vi "ModeDrivebase.vi"(0 "Master State":enum16{"Normal", "Climb"}(ring)) -> (1 "Drive Mode Change":bool, 2 "Drive Mode":T1(ring))   [LabVIEW 2020]
doc: "This VI manages the robot drivebase mode. The default mode is driver control in which the swerve drive accepts all drive inputs and seemlessly combines them with autonomous heading corrections. Two auto targeting modes are also implimented."
uses:
  dscommands.vi
  dsdata.vi
  sensors.vi
  outputs.vi
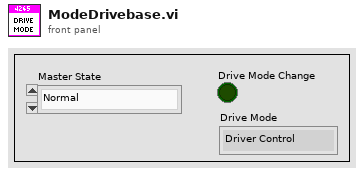
[diagram p1: front panel]
types:
  T1 = enum16{"Driver Control", "Auto Targeting", "Feeder Station"}
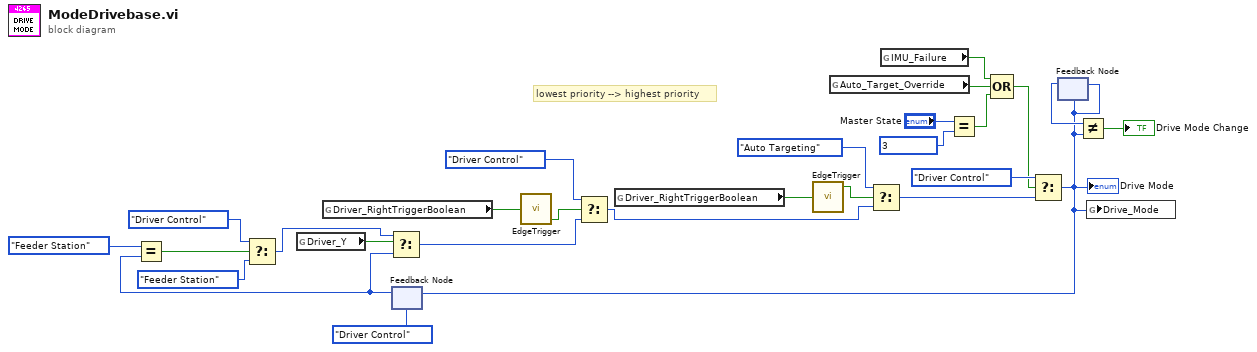
[diagram p0: block diagram]
diagram:
  # "lowest priority --> highest priority"
  n1 = global read "dscommands.vi" "Driver_Y"() -> (w14:bool)
  n2 = global read "dscommands.vi" "Driver_RightTriggerBoolean"() -> (w6:bool)
  n3 = feedback #1(T1."Driver Control") -> (w11:T1)
  n4 = Equal?(x=T1."Feeder Station", y=w11) -> (x = y?=w19:bool)
  n5 = Select(t=T1."Driver Control", s=w19, f=T1."Feeder Station") -> (s? t:f=w8:T1)
  n6 = Select(t=w8, s=w14, f=w11) -> (s? t:f=w4:T1)
  n7 = call "EdgeTrigger.vi"("Input Signal"=w6) -> ("Falling Edge Trigger"=w5:bool)  [unwired: 2 out]
  n8 = Select(t=T1."Driver Control", s=w5, f=w4) -> (s? t:f=w3:T1)
  n9 = global read "dscommands.vi" "Driver_RightTriggerBoolean"() -> (w10:bool)
  n10 = call "EdgeTrigger.vi"("Input Signal"=w10) -> ("Rising Edge Trigger"=w9:bool)  [unwired: 2 out]
  n11 = global read "dsdata.vi" "Auto_Target_Override"() -> (w13:bool)
  n12 = Select(t=T1."Auto Targeting", s=w9, f=w3) -> (s? t:f=w24:T1)
  n13 = global read "sensors.vi" "IMU_Failure"() -> (w12:bool)
  n14 = Equal?(x="Master State", y=enum16{"Normal", "Climb"} 3) -> (x = y?=w16:bool)
  n15 = Compound Arithmetic op=OR(w12, w13, w16) -> (w15:bool)
  n16 = Select(t=T1."Driver Control", s=w15, f=w24) -> (s? t:f=w22:T1)
  "Drive Mode" <- w22
  n17 = feedback-in #1(w22) -> ()
  n18 = feedback #2(w22) -> (w26:T1)
  n19 = feedback-in #2(w22) -> ()
  n20 = Not Equal?(x=w26, y=w22) -> (x != y?=→"Drive Mode Change":bool)
  n21 = global write "outputs.vi" "Drive_Mode"(w22) -> ()
